vi "GetGEA2HyperData.vi"(0 "ComPort":refnum<visa-resource-name>="COM1", 5 "Retry":i32, 11 "Error In":errorcluster) -> (4 "CRC":bool, 6 "GEA2 Hyperdata":string, 15 "Error Out":errorcluster)   [LabVIEW 2009]
uses:
  <vilib>/Utility/error.llb/whitespace.ctl
  HEWH Command Type.ctl
  Global HEWH.vi
panel:
  out "appended array":string[][](array[string])
  out "DataReturned":u8[](array[numeric])
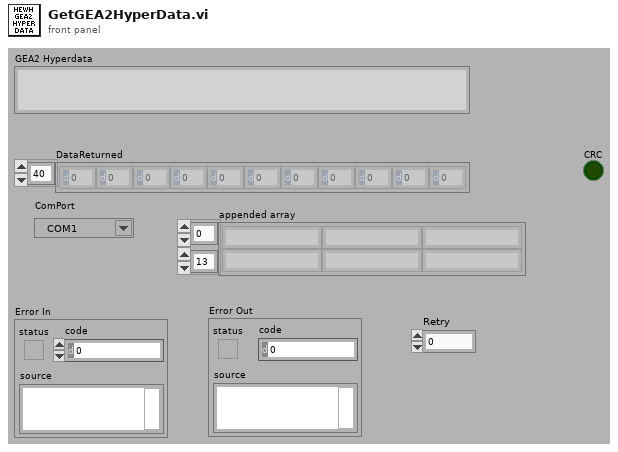
[diagram p1: front panel]
types:
  T1 = typedef "HEWH Command Type.ctl" = u8
  T2 = typedef "whitespace.ctl" = u16
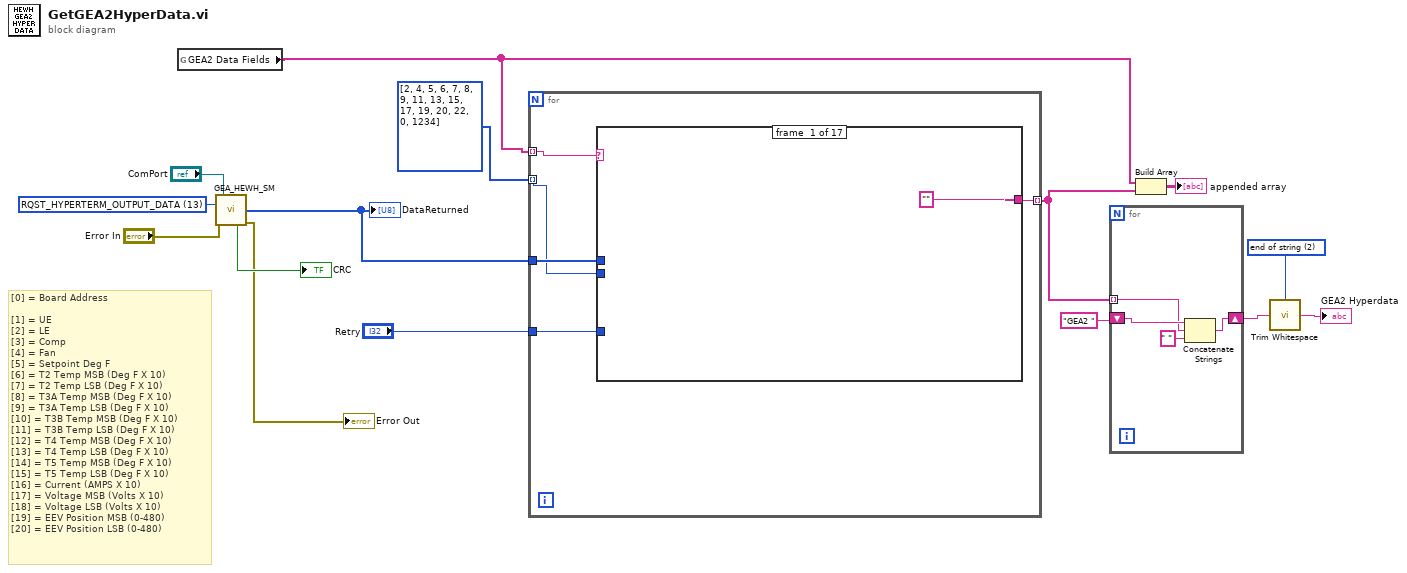
[diagram p0: block diagram]
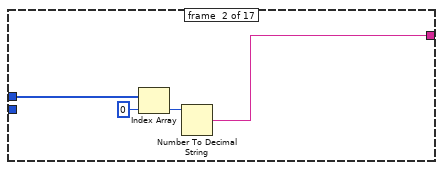
[diagram p2: hidden frame]
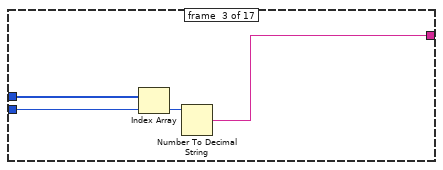
[diagram p3: hidden frame]
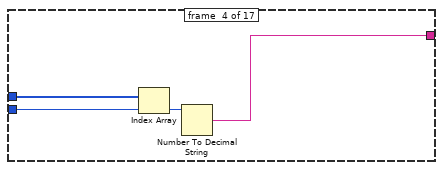
[diagram p4: hidden frame]
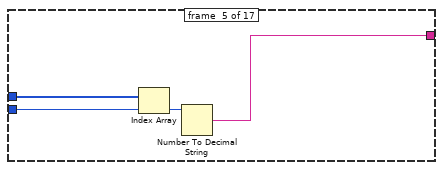
[diagram p5: hidden frame]
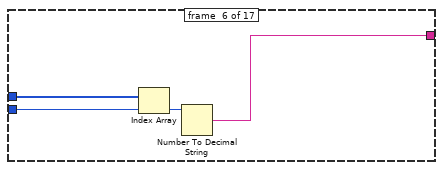
[diagram p6: hidden frame]
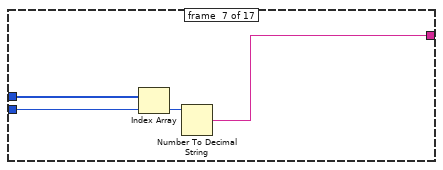
[diagram p7: hidden frame]
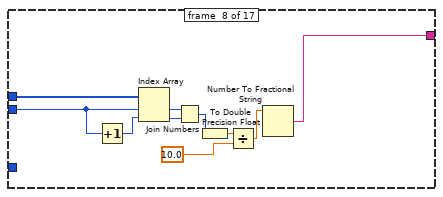
[diagram p8: hidden frame]
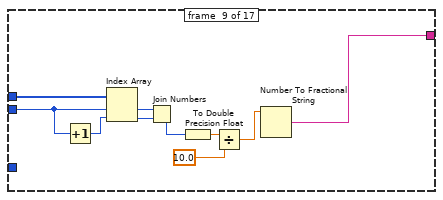
[diagram p9: hidden frame]
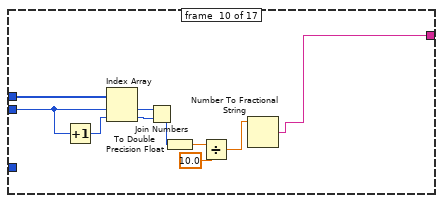
[diagram p10: hidden frame]
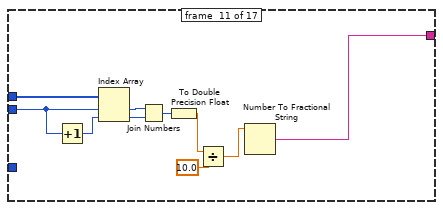
[diagram p11: hidden frame]
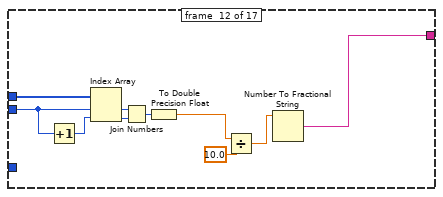
[diagram p12: hidden frame]
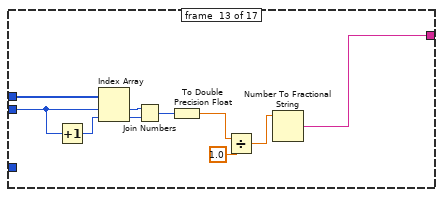
[diagram p13: hidden frame]
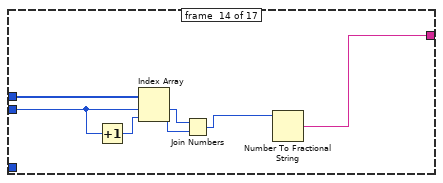
[diagram p14: hidden frame]
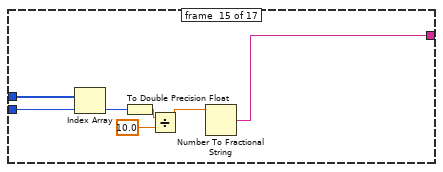
[diagram p15: hidden frame]
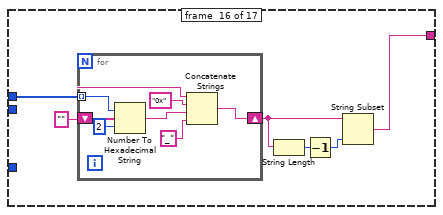
[diagram p16: hidden frame]
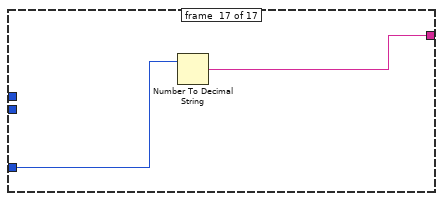
[diagram p17: hidden frame]
diagram:
  w1 = T1 13 items=["RQST_SOFTWARE_VERSION", "RQST_T2_RESISTANCE", "RQST_T3A_RESISTANCE", "RQST_T3B_RESISTANCE", "RQST_T4_RESISTANCE", "RQST_T5_RESISTANCE", "RQST_IDLB_RESISTANCE", "RQST_MODE_SELECT_RESISTANCE", "RQST_DATA_FROM_MEMORY", "RQST_DATA_FROM_DATA_FLASH", "RQST_SS_FAULT_COUNTS", "RQST_OTHER_FAULT_COUNTS", "CMD_CLEAR_FAULT_COUNTS", "RQST_HYPERTERM_OUTPUT_DATA", "CMD_RESET_FILTER_TIMES", "CMD_WRITE_SETPOINTS", "CMD_TURN_ON_OFF_DLB", "CMD_ENTER_EXIT_FCT_MODE", "CMD_SET_LEDS", "CMD_SET_EEV_DRIVE_LINES", "REQ_READ_KEY_STATUS", "RQST_READ_PERSONALITY", "CMD_ENTER_FACT_MODE", "CMD_RESET", "CMD_RESTORE_EEPROM_DEFAULTS", "CMD_SET_MODEL_NUMBER", "CMD_SET_SERIAL_NUMBER", "RQST_MODEL_NUMBER", "RQST_SERIAL_NUMBER", "CMD_TOGGLE_SERVICE_MODE", "CMD_TOGGLE_UE_SERV", "CMD_TOGGLE_LE_SERV", "CMD_REFRESH_SERVICE_TIMEOUTS", "RQST_DSM_OVERRIDE_STATUS", "RQST_STATUS_QUERY", "RQST_HEM_KWH_DATA", "RQST_SERVICE_ERROR_CODES", "RQST_OVERRIDE_STATUS", "CMD_UPDATE_DSM_LEVEL", "CMD_OVERRIDE_STATUS_CHANGED", "CMD_CLEAR_OVERRIDE_STATUS", "CMD_CLEAR_ENERGY_USAGE_CTRS", "CMD_DSM_OVERRIDES", "CMD_UPDATE_MODE", "CMD_SET_PID_P_DENOMINATOR", "CMD_SET_PID_I_DENOM_UNDER_THR", "CMD_SET_PID_I_DENOM_OVER_THR", "CMD_SET_START_POS_UNDER_THR", "CMD_SET_START_POS_OVER_THR", "CMD_SET_EEV_STOP_POSITION", "CMD_SET_AMBIENT_THRESH_1", "CMD_SET_AMBIENT_THRESH_2", "CMD_SET_AMBIENT_THRESH_3", "CMD_SET_PID_LOW_SH_TARGET", "CMD_SET_PID_MID_SH_TARGET", "RQST_PID_PARAMETERS", "CMD_COMP_OFF", "CMD_TOGGLE_FAN", "CMD_RQST_LED_STATUS", "CMD_UE_2_SECONDS", "CMD_LE_2_SECONDS", "CMD_COMP_ON", "CMD_HP_RUN_6MIN", "RQST_TEMP_RANGE", "RQST_VACATION_RANGE", "RQST_STD_ELEC_RANGE", "RQST_WATER_CAPACITY", "CMD_CANCEL_EEV_POSITION", "CMD_EEV_POSITION", "CMD_SET_CURRENTS", "RQST_SUPPORTED_MODES"] ("Command")
  w7 = T2 2 items=["both", "start of string", "end of string"] ("location (both)")
  # "[0] = Board Address\n\n[1] = UE\n[2] = LE\n[3] = Comp\n[4] = Fan\n[5] = Setpoint Deg F\n[6] = T2 Temp MSB (Deg F X 10)\n[7] = T2 Temp LSB (Deg F X 10)\n[8] = T3A Temp MSB (Deg F X 10)\n[9] = T3A Temp LSB (Deg F X 10)\n[10] = T3B Temp MSB (Deg F X 10)\n[11] = T3B Temp LSB (Deg F X 10)\n[12] = T4 Temp MSB (Deg F X 10)\n[13] = T4 Temp LSB (Deg F X 10)\n[14] = T5 Temp MSB (Deg F X 10)\n[15] = T5 Temp LSB (Deg F X 10)\n[16] = Current (AMPS X 10)\n[17] = Voltage MSB (Volts X 10)\n[18] = Voltage LSB (Volts X 10)\n[19] = EEV Position MSB (0-480)\n[20] = EEV Position LSB (0-480)"
  n1 = global read "Global HEWH.vi" "GEA2 Data Fields"() -> (w3:string[])
  n2 = call "GEA_HEWH_SM.vi"("ComPort"="ComPort", "Command"=w1, "Error In"="Error In") -> ("DataReturned"=w5:u8[], "CRC Match"=→"CRC":bool, "Error Out"=→"Error Out":errorcluster)  [unwired: 8 in, 2 out]
  "DataReturned" <- w5
  n3 = for {
    tunnel: w3 -> [w20] mode=indexing
    tunnel: w5 -> [w19]
    tunnel: [w18] -> w11 mode=indexing
    tunnel: i32[] [2, 4, 5, 6, 7, 8, 9, 11, 13, 15, 17, 19, 20, 22, 0, 1234] -> [w17] mode=indexing
    tunnel: "Retry" -> [w16]
    n4 = case shown="\"Com Err Count\"" w20 {
      tunnel: w19 -> [_ w25 w29 w33 w37 w41 w45 w55 w65 w75 w85 w95 w105 w112 w119 w125 _]
      tunnel: ["" w22 w27 w31 w35 w39 w43 w54 w57 w67 w77 w87 w97 w107 w118 w120 w133] -> w18
      tunnel: w17 -> [_ _ w26 w30 w34 w38 w42 w52 w63 w73 w83 w93 w103 w110 w117 _ _]
      tunnel: w16 -> [_ _ _ _ _ _ _ _ _ _ _ _ _ _ _ _ w134]
      frame #0 {
      }
      frame #1 {
        n5 = Index Array(array=w25, index=0) -> (element=w23:u8)
        n6 = Number To Decimal String(number=w23) -> (decimal integer string=w22:string)  [unwired: 1 in]
      }
      frame #2 {
        n7 = Index Array(array=w29, index=w26) -> (element=w28:u8)
        n8 = Number To Decimal String(number=w28) -> (decimal integer string=w27:string)  [unwired: 1 in]
      }
      frame #3 {
        n9 = Index Array(array=w33, index=w30) -> (element=w32:u8)
        n10 = Number To Decimal String(number=w32) -> (decimal integer string=w31:string)  [unwired: 1 in]
      }
      frame #4 {
        n11 = Index Array(array=w37, index=w34) -> (element=w36:u8)
        n12 = Number To Decimal String(number=w36) -> (decimal integer string=w35:string)  [unwired: 1 in]
      }
      frame #5 {
        n13 = Index Array(array=w41, index=w38) -> (element=w40:u8)
        n14 = Number To Decimal String(number=w40) -> (decimal integer string=w39:string)  [unwired: 1 in]
      }
      frame #6 {
        n15 = Index Array(array=w45, index=w42) -> (element=w44:u8)
        n16 = Number To Decimal String(number=w44) -> (decimal integer string=w43:string)  [unwired: 1 in]
      }
      frame #7 {
        n17 = Increment(x=w52) -> (x+1=w53:i32)
        n18 = Index Array(array=w55, index #1=w52, index #2=w53) -> (element #1=w51:u8, element #2=w50:u8)
        n19 = Join Numbers(hi=w51, lo=w50) -> ((hi.lo)=w49:u16)
        n20 = To Double Precision Float(number=w49) -> (double precision float=w46:dbl)
        n21 = Divide(x=w46, y=10.0) -> (x/y=w47:dbl)
        n22 = Number To Fractional String(number=w47) -> (F-format string=w54:string)  [unwired: 3 in]
      }
      frame #8 {
        n23 = Increment(x=w63) -> (x+1=w64:i32)
        n24 = Index Array(array=w65, index #1=w63, index #2=w64) -> (element #1=w62:u8, element #2=w61:u8)
        n25 = Join Numbers(hi=w62, lo=w61) -> ((hi.lo)=w58:u16)
        n26 = To Double Precision Float(number=w58) -> (double precision float=w56:dbl)
        n27 = Divide(x=w56, y=10.0) -> (x/y=w59:dbl)
        n28 = Number To Fractional String(number=w59) -> (F-format string=w57:string)  [unwired: 3 in]
      }
      frame #9 {
        n29 = Increment(x=w73) -> (x+1=w74:i32)
        n30 = Index Array(array=w75, index #1=w73, index #2=w74) -> (element #1=w72:u8, element #2=w71:u8)
        n31 = Join Numbers(hi=w72, lo=w71) -> ((hi.lo)=w68:u16)
        n32 = To Double Precision Float(number=w68) -> (double precision float=w66:dbl)
        n33 = Divide(x=w66, y=10.0) -> (x/y=w69:dbl)
        n34 = Number To Fractional String(number=w69) -> (F-format string=w67:string)  [unwired: 3 in]
      }
      frame #10 {
        n35 = Increment(x=w83) -> (x+1=w84:i32)
        n36 = Index Array(array=w85, index #1=w83, index #2=w84) -> (element #1=w82:u8, element #2=w81:u8)
        n37 = Join Numbers(hi=w82, lo=w81) -> ((hi.lo)=w78:u16)
        n38 = To Double Precision Float(number=w78) -> (double precision float=w76:dbl)
        n39 = Divide(x=w76, y=10.0) -> (x/y=w79:dbl)
        n40 = Number To Fractional String(number=w79) -> (F-format string=w77:string)  [unwired: 3 in]
      }
      frame #11 {
        n41 = Increment(x=w93) -> (x+1=w94:i32)
        n42 = Index Array(array=w95, index #1=w93, index #2=w94) -> (element #1=w92:u8, element #2=w91:u8)
        n43 = Join Numbers(hi=w92, lo=w91) -> ((hi.lo)=w88:u16)
        n44 = To Double Precision Float(number=w88) -> (double precision float=w86:dbl)
        n45 = Divide(x=w86, y=10.0) -> (x/y=w89:dbl)
        n46 = Number To Fractional String(number=w89) -> (F-format string=w87:string)  [unwired: 3 in]
      }
      frame #12 {
        n47 = Increment(x=w103) -> (x+1=w104:i32)
        n48 = Index Array(array=w105, index #1=w103, index #2=w104) -> (element #1=w102:u8, element #2=w101:u8)
        n49 = Join Numbers(hi=w102, lo=w101) -> ((hi.lo)=w98:u16)
        n50 = To Double Precision Float(number=w98) -> (double precision float=w96:dbl)
        n51 = Divide(x=w96, y=1.0) -> (x/y=w99:dbl)
        n52 = Number To Fractional String(number=w99) -> (F-format string=w97:string)  [unwired: 3 in]
      }
      frame #13 {
        n53 = Increment(x=w110) -> (x+1=w111:i32)
        n54 = Index Array(array=w112, index #1=w110, index #2=w111) -> (element #1=w109:u8, element #2=w108:u8)
        n55 = Join Numbers(hi=w109, lo=w108) -> ((hi.lo)=w106:u16)
        n56 = Number To Fractional String(number=w106) -> (F-format string=w107:string)  [unwired: 3 in]
      }
      frame #14 {
        n57 = Index Array(array=w119, index=w117) -> (element=w116:u8)
        n58 = To Double Precision Float(number=w116) -> (double precision float=w113:dbl)
        n59 = Divide(x=w113, y=10.0) -> (x/y=w115:dbl)
        n60 = Number To Fractional String(number=w115) -> (F-format string=w118:string)  [unwired: 3 in]
      }
      frame #15 {
        n61 = for {
          tunnel: w125 -> [w132] mode=indexing
          shift-right: [w130] -> w121
          shift-left: "" -> [w128]
          n62 = Number To Hexadecimal String(1:i16 2 ("width (-)"), 2:w132) -> (0:w131:string)
          n63 = Concatenate Strings(w128, "0x" ("string"), w131, "_" ("string")) -> (w130:string)
        }
        n64 = String Length(string=w121) -> (length=w123:i32)
        n65 = Decrement(x=w123) -> (x-1=w122:i32)
        n66 = String Subset(string=w121, length (rest)=w122) -> (substring=w120:string)  [unwired: 1 in]
      }
      frame #16 {
        n67 = Number To Decimal String(number=w134) -> (decimal integer string=w133:string)  [unwired: 1 in]
      }
    }
  }
  n68 = for {
    tunnel: w11 -> [w137] mode=indexing
    shift-right: [w135] -> w9
    shift-left: "GEA2 " -> [w138]
    n69 = Concatenate Strings(w138, w137, " " ("string")) -> (w135:string)
  }
  n70 = Build Array(w3, w11) -> (→"appended array":string[][])
  n71 = call <vilib>:"Trim Whitespace.vi"("string"=w9, "location (both)"=w7) -> ("trimmed string"=→"GEA2 Hyperdata":string)
